vi "Detect Digital Audio HW.vi"(8 "error in (no error)":errorcluster) -> (0 "error out":errorcluster, 3 "alias":string[](array[string]))   [LabVIEW 2021, in "AudioGenUtility.lvlib"]
uses:
  AudioGenUtility.lvlib
  <vilib>/nisyscfg/Close (System).vi
  <vilib>/nisyscfg/nisyscfg.lvlib
  <resource>/objmgr/niflexrioatomicsae.rc
  <resource>/objmgr/nicontrollersysapi.rc
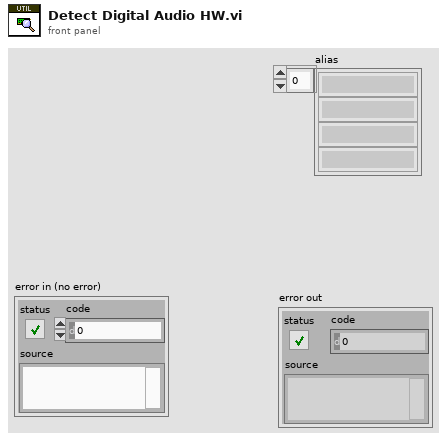
[diagram p1: front panel]
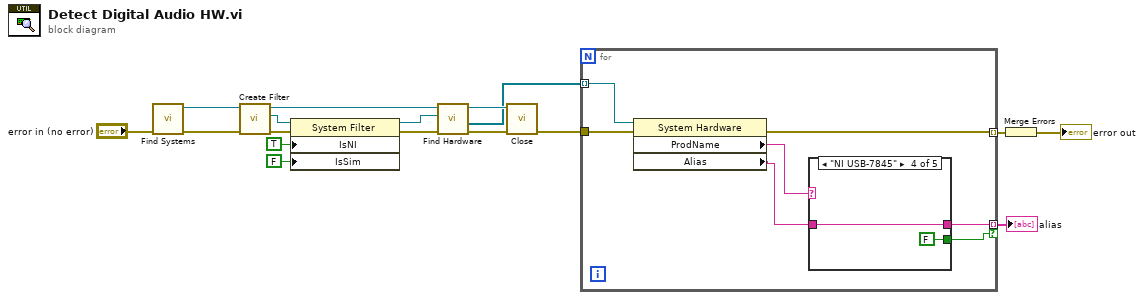
[diagram p0: block diagram]
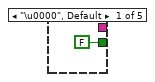
[diagram p2: hidden frame]
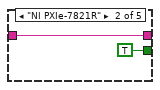
[diagram p3: hidden frame]
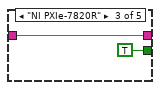
[diagram p4: hidden frame]
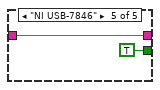
[diagram p5: hidden frame]
diagram:
  n1 = call <vilib>:"Find Systems.vi"("error in (no error)"="error in (no error)") -> ("error out"=w14:errorcluster, "Session out"=w15:refnum<k21>)  [unwired: 8 in, 1 out]
  n2 = call <vilib>:"Create Filter.vi"("error in (no error)"=w14, "Session in"=w15) -> ("error out"=w17:errorcluster, "Filter out"=w16:refnum<k20>, "Session out"=w9:refnum<k21>)  [unwired: 7 in]
  n3 = property class="System Filter"(reference=w16, error in=w17, "IsNI"=TRUE ("Devices & Chassis:Is NI Product"), "IsSim"=FALSE ("Devices & Chassis:Is Simulated")) -> (reference out=w10:refnum<k20>, error out=w11:errorcluster)
  n4 = call <vilib>:"Find Hardware.vi"("error in (no error)"=w11, "Filter in"=w10, "Session in"=w9) -> ("error out"=w7:errorcluster, "Resources out"=w6:refnum<k20>[], "Session out"=w8:refnum<k21>)  [unwired: 5 in, 1 out]
  n5 = call-poly <vilib>:"Close.vi"("error in (no error)"=w7, "Session in"=w8) -> ("error out"=w5:errorcluster)  [unwired: 9 in]
  n6 = for {
    tunnel: w6 -> [w23] mode=indexing
    tunnel: w5 -> [w24]
    tunnel: [w22] -> w4 mode=indexing
    tunnel: [w19] -> w3 mode=indexing if=w18
    n7 = property class="System Hardware"(reference=w23, error in=w24) -> (error out=w22:errorcluster, "ProdName"=w21:string, "Alias"=w20:string)  [unwired: 1 out]
    n8 = case shown="\"NI USB-7845\"" w21 {
      tunnel: w20 -> [_ w27 w29 w31 w33]
      tunnel: [_ w27 w29 w31 w33] -> w19
      tunnel: [FALSE TRUE TRUE FALSE TRUE] -> w18
      frame "\u0000", Default {
      }
      frame "NI PXIe-7821R" {
      }
      frame "NI PXIe-7820R" {
      }
      frame "NI USB-7845" {
      }
      frame "NI USB-7846" {
      }
    }
  }
  "alias" <- w3
  n9 = Merge Errors(w4) -> (→"error out":errorcluster)
